vi "Dpc End Notify.vi"(8 "error in (no error)":errorcluster, 10 "perc":i32, 11 "hwndTemp":u32) -> (0 "error out":errorcluster, 1 "function return":i32, 2 "perc out":i32, 3 "hwndTemp out":u32)   [LabVIEW 2011, in "LVH-Adept.lvlib" / "DPCUTIL.lvlib"]
doc: "DPCAPI BOOL DpcEndNotify(HWND hwndTemp, ERC *perc);"
uses:
  DPCUTIL.lvlib
  Resources/dpcutil.dll
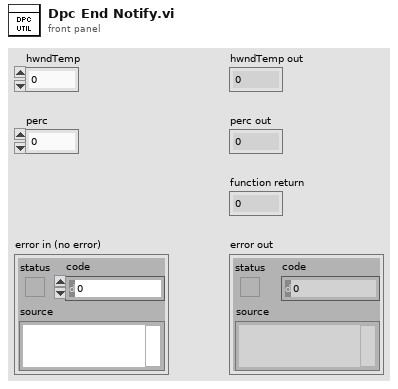
[diagram p1: front panel]
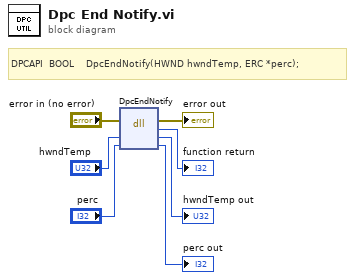
[diagram p0: block diagram]
diagram:
  # "DPCAPI  BOOL    DpcEndNotify(HWND hwndTemp, ERC *perc);"
  n1 = dll-call lib="C:/github/labviewhacker/LVH-Adept/LabVIEW/vi.lib/LabVIEW Hacker/Adept/Private/Resources/dpcutil.*" fn="DpcEndNotify"(error in="error in (no error)", "hwndTemp"="hwndTemp", "perc"="perc") -> (error out=→"error out":errorcluster, →"function return":i32, "hwndTemp"=→"hwndTemp out":u32, "perc"=→"perc out":i32)  [unwired: 2 in, 1 out]
